vi "Get Active Target Hostname.vi"(8 "error in":errorcluster) -> (0 "error out":errorcluster, 3 "IP Address / Hostname":string)   [LabVIEW 2020, in "Scan Engine EtherCAT System Tests.lvclass"]
uses:
  Scan Engine EtherCAT System Tests.lvclass
  <vilib>/NI/VeriStand Custom Device Testing Tools/VeriStandTestUtilities/VeriStandTestUtilities.lvlib
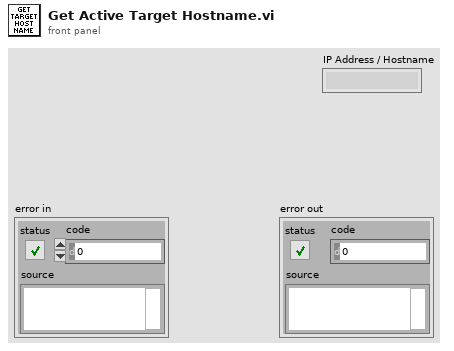
[diagram p1: front panel]
types:
  T1 = typedef "VeriStandTestUtilities.lvlib/TargetsConfiguration.ctl" = cluster{"Supported Targets":cluster{"IP Address / Hostname":string, "Target Platform":T2}[], "Active Configuration":T2}
  T2 = typedef "VeriStandTestUtilities.lvlib/TargetPlatform.ctl" = enum16{"Windows", "Linux64CRIO", "Linux64PXI", "LinuxARM", "PharLap"}
  T3 = cluster{"IP Address / Hostname":string, "Target Platform":T2}[]
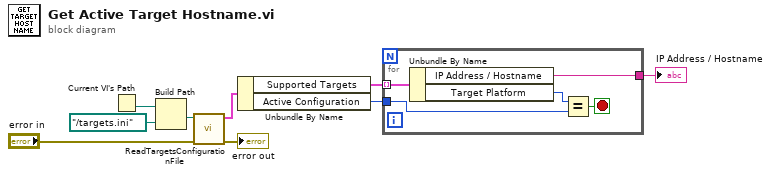
[diagram p0: block diagram]
diagram:
  n1 = Current VI's Path() -> (path=w4:path)
  n2 = Build Path(base path=w4, name or relative path=path "../targets.ini") -> (appended path=w6:path)
  n3 = call <vilib>:"ReadTargetsConfigurationFile.vi"("error in (no error)"="error in", "targets.ini file"=w6) -> ("error out"=→"error out":errorcluster, "Targets Configuration"=w7:T1)  [unwired: 8 in]
  n4 = Unbundle By Name(w7) -> ("Supported Targets"=w8:T3, "Active Configuration"=w9:T2)
  n5 = for {
    tunnel: w8 -> [w14] mode=indexing
    tunnel: w9 -> [w12]
    tunnel: [w10] -> w1
    stop <- w11 stop-if-true
    n6 = Unbundle By Name(w14) -> ("IP Address / Hostname"=w10:string, "Target Platform"=w13:T2)
    n7 = Equal?(x=w13, y=w12) -> (x = y?=w11:bool)
  }
  "IP Address / Hostname" <- w1
